vi "Initialise.vi"(8 "error in (no error)":errorcluster, 10 "Init":T1, 11 "Cube in":refnum<class "Cube.lvclass">) -> (0 "error out":errorcluster, 3 "Cube out":refnum<class "Cube.lvclass">)   [LabVIEW 2019, in "22.lvlib" / "Cube.lvclass"]
uses:
  Cube.lvclass
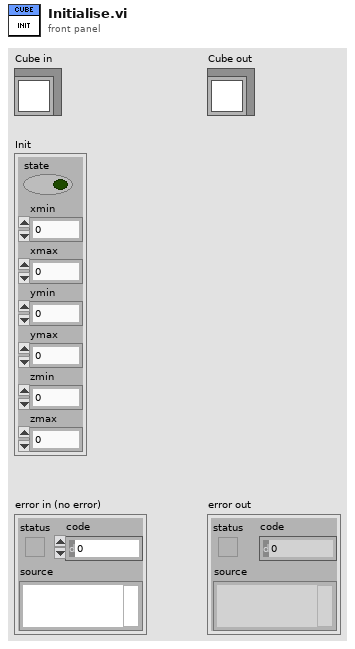
[diagram p1: front panel]
types:
  T1 = cluster{"state":bool, "xmin":i64, "xmax":i64, "ymin":i64, "ymax":i64, "zmin":i64, "zmax":i64}
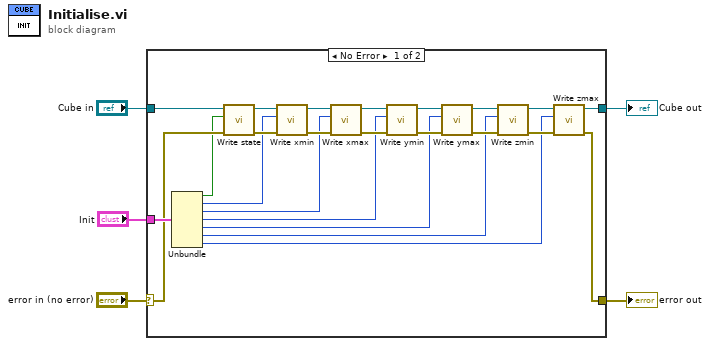
[diagram p0: block diagram]
diagram:
  n1 = case shown="No Error" "error in (no error)" {
    selector: "error in (no error)" -> [w14 w31]
    tunnel: [w13 w31] -> w4
    tunnel: [w19 w30] -> w2
    tunnel: "Cube in" -> [w16 w30]
    tunnel: "Init" -> [w26 _]
    frame No Error {
      n2 = Unbundle(w26) -> ("state"=w12:bool, "xmin"=w11:i64, "xmax"=w10:i64, "ymin"=w9:i64, "ymax"=w8:i64, "zmin"=w7:i64, "zmax"=w6:i64)
      n3 = call-dynamic "Write state.vi"("error in (no error)"=w14, "state"=w12, "Cube in"=w16) -> ("error out"=w15:errorcluster, "Cube out"=w17:refnum<class "Cube.lvclass">)  [unwired: 7 in]
      n4 = call-dynamic "Write xmin.vi"("error in (no error)"=w15, "xmin"=w11, "Cube in"=w17) -> ("error out"=w28:errorcluster, "Cube out"=w29:refnum<class "Cube.lvclass">)  [unwired: 7 in]
      n5 = call-dynamic "Write xmax.vi"("error in (no error)"=w28, "xmax"=w10, "Cube in"=w29) -> ("error out"=w25:errorcluster, "Cube out"=w27:refnum<class "Cube.lvclass">)  [unwired: 7 in]
      n6 = call-dynamic "Write ymin.vi"("error in (no error)"=w25, "ymin"=w9, "Cube in"=w27) -> ("error out"=w23:errorcluster, "Cube out"=w24:refnum<class "Cube.lvclass">)  [unwired: 7 in]
      n7 = call-dynamic "Write ymax.vi"("error in (no error)"=w23, "ymax"=w8, "Cube in"=w24) -> ("error out"=w21:errorcluster, "Cube out"=w22:refnum<class "Cube.lvclass">)  [unwired: 7 in]
      n8 = call-dynamic "Write zmin.vi"("error in (no error)"=w21, "zmin"=w7, "Cube in"=w22) -> ("error out"=w18:errorcluster, "Cube out"=w20:refnum<class "Cube.lvclass">)  [unwired: 7 in]
      n9 = call-dynamic "Write zmax.vi"("error in (no error)"=w18, "zmax"=w6, "Cube in"=w20) -> ("error out"=w13:errorcluster, "Cube out"=w19:refnum<class "Cube.lvclass">)  [unwired: 7 in]
    }
    frame Error {
    }
  }
  "error out" <- w4
  "Cube out" <- w2
